vi "DateString2TimeStamp.vi"(4 "DateString(YYYY/MM/DD)":string) -> (1 "time stamp":timestamp)   [LabVIEW 2022 SP3]
uses:
  <vilib>/Utility/miscctls.llb/LVDateTimeRec.ctl
panel:
  in  "DateFormat":enum16{"YYYY/MM/DD", "MM/DD/YYYY", "DD/MM/YYYY"}(ring)
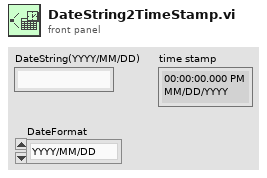
[diagram p1: front panel]
types:
  T1 = typedef "LVDateTimeRec.ctl" = cluster{"fractional second":dbl, "second":i32, "minute":i32, "hour":i32, "day of month":i32, "month":i32, "year":i32, "day of week":i32, "day of year":i32, "DST":i32}
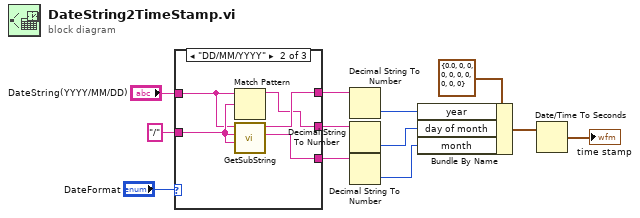
[diagram p0: block diagram]
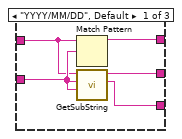
[diagram p2: hidden frame]
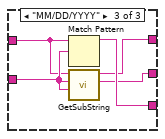
[diagram p3: hidden frame]
diagram:
  n1 = case shown="\"DD/MM/YYYY\"" "DateFormat" {
    tunnel: [w17 w18 w25] -> w6
    tunnel: [w16 w19 w23] -> w5
    tunnel: [w15 w20 w24] -> w4
    tunnel: "/" ("Start Search") -> [w14 w22 w27]
    tunnel: "DateString(YYYY/MM/DD)" -> [w13 w21 w26]
    frame "YYYY/MM/DD", Default {
      n2 = Match Pattern(string=w13, regular expression=w14) -> (before substring=w15:string)  [unwired: 1 in, 3 out]
      n3 = call "GetSubString.vi"("End Search"=w14, "Start Search"=w14, "String In"=w13) -> ("Match"=w17:string, "Following String Out"=w16:string)  [unwired: 6 in, 1 out]
    }
    frame "DD/MM/YYYY" {
      n4 = Match Pattern(string=w21, regular expression=w22) -> (before substring=w19:string)  [unwired: 1 in, 3 out]
      n5 = call "GetSubString.vi"("End Search"=w22, "Start Search"=w22, "String In"=w21) -> ("Match"=w18:string, "Following String Out"=w20:string)  [unwired: 6 in, 1 out]
    }
    frame "MM/DD/YYYY" {
      n6 = Match Pattern(string=w26, regular expression=w27) -> (before substring=w25:string)  [unwired: 1 in, 3 out]
      n7 = call "GetSubString.vi"("End Search"=w27, "Start Search"=w27, "String In"=w26) -> ("Match"=w23:string, "Following String Out"=w24:string)  [unwired: 6 in, 1 out]
    }
  }
  n8 = Decimal String To Number(string=w4) -> (number=w9:i32)  [unwired: 2 in, 1 out]
  n9 = Decimal String To Number(string=w5) -> (number=w10:i32)  [unwired: 2 in, 1 out]
  n10 = Decimal String To Number(string=w6) -> (number=w11:i32)  [unwired: 2 in, 1 out]
  n11 = Bundle By Name(cluster=T1 {"fractional second"=0.0, "second"=0, "minute"=0, "hour"=0, "day of month"=0, "month"=0, "year"=0, "day of week"=0, "day of year"=0, "DST"=0} ("date time rec"), "year"=w9, "day of month"=w10, "month"=w11) -> (w8:T1)
  n12 = Date/Time To Seconds(2:w8) -> (0:→"time stamp":timestamp)  [unwired: 1 in]
